vi "Read View.vi"(8 "error in (no error)":errorcluster, 11 "View Test In":refnum<class "View Test.lvclass">) -> (0 "error out":errorcluster, 2 "View":refnum<class "View.lvclass">, 3 "View Test Out":refnum<class "View Test.lvclass">)   [LabVIEW 2020, in "View Test.lvclass"]
uses:
  View Test.lvclass
  Framework/View/View.lvclass
  C:/Users/anton/Documents/GitHub/Triarc-Framework/source/Framework Test/Base Class Test/Base Test.lvclass
  Base Class Test/Base Test.lvclass/Base Test.ctl
  Framework/Base/Base.lvclass
  Base Class Test/Base Test.lvclass
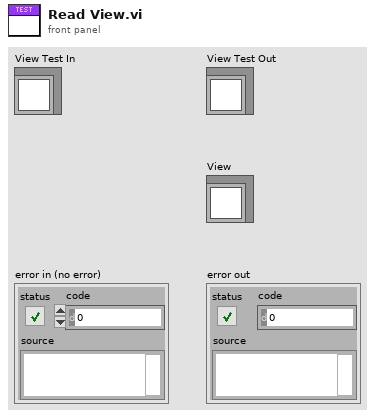
[diagram p1: front panel]
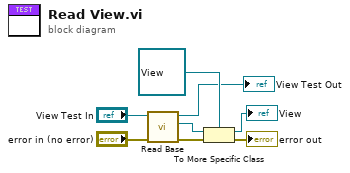
[diagram p0: block diagram]
diagram:
  n1 = call "Read Base.vi"("error in (no error)"="error in (no error)", "Base Class Test In"="View Test In") -> ("error out"=w5:errorcluster, "Base.lvclass"=w4:refnum<class "Base.lvclass">, "Base Class Test Out"=→"View Test Out":refnum<class "View Test.lvclass">)  [unwired: 7 in]
  n2 = To More Specific Class(target class=refnum<class "View.lvclass"> refnum ("UI View.lvclass"), reference=w4, error in=w5) -> (specific class reference=→"View":refnum<class "View.lvclass">, error out=→"error out":errorcluster)
